vi "synth generation.vi"(8 "error in (no error)":errorcluster, 11 "Refnum in":T1) -> (0 "error out":errorcluster, 3 "Refnum out":T1)   [LabVIEW 2014]
uses:
  Controls/FPGA Reference.ctl
  Controls/ADSR State.ctl
  Controls/Application Data.vi
  <vilib>/Utility/error.llb/Error Cluster From Error Code.vi
  <vilib>/rvi/errors/niLvFpgaAdjustHostInterfaceError.vi
  <vilib>/rvi/interface/nirviMethod/nirviMethod.xnode
  <vilib>/FPGAPlugInAG/Dynamic/niLvFpga_WriteFifo_Dynamic.vi
  <vilib>/rvi/errors/niLvFpgaMergeErrorWithErrorCode.vi
panel:
  in  "Attack (ms) 2":dbl=1000.0
  in  "Max. Amplitude (V) 2":dbl(slide)=0.7993311036789298 scale=0.0..1.0
  in  "Sustain  2":dbl=0.6
  in  "Decay (ms) 2":dbl=300.0
  in  "Sustain 2":dbl=300.0
  in  "Release":dbl=300.0
  out "Gain2":dbl
  out "Gain Graph 2":dbl(graph)
  out "Waveform Chart":dbl[](graph)
  in  "Y":dbl[](array[numeric])
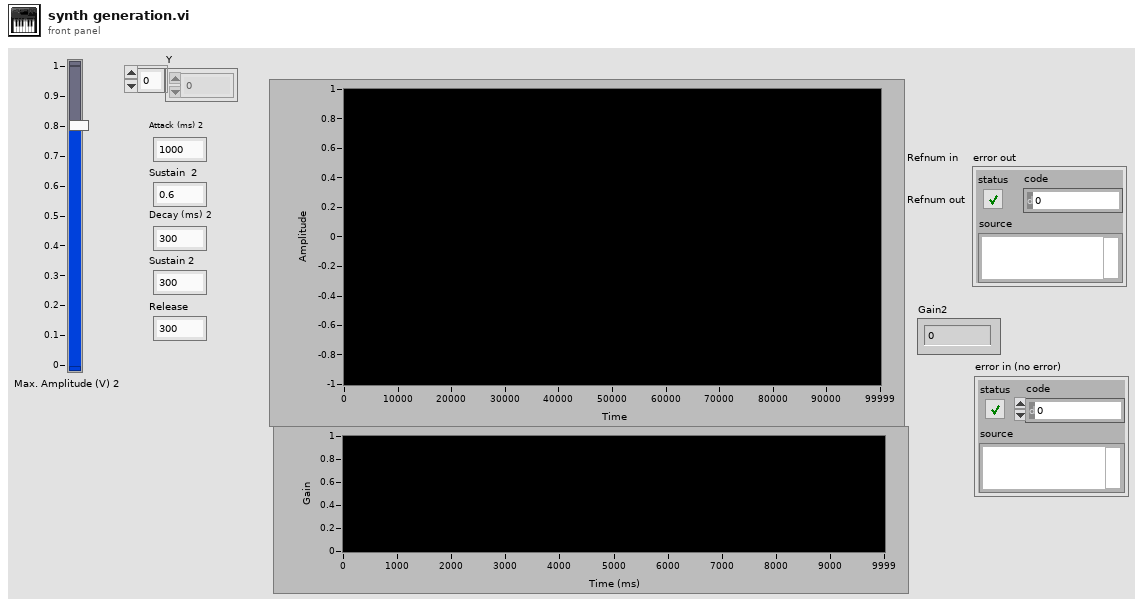
[diagram p1: front panel]
types:
  T1 = typedef "FPGA Reference.ctl" = refnum<k20>
  T2 = typedef "ADSR State.ctl" = enum16{"Attack", "Decay", "Sustain", "Release", "Idle"}
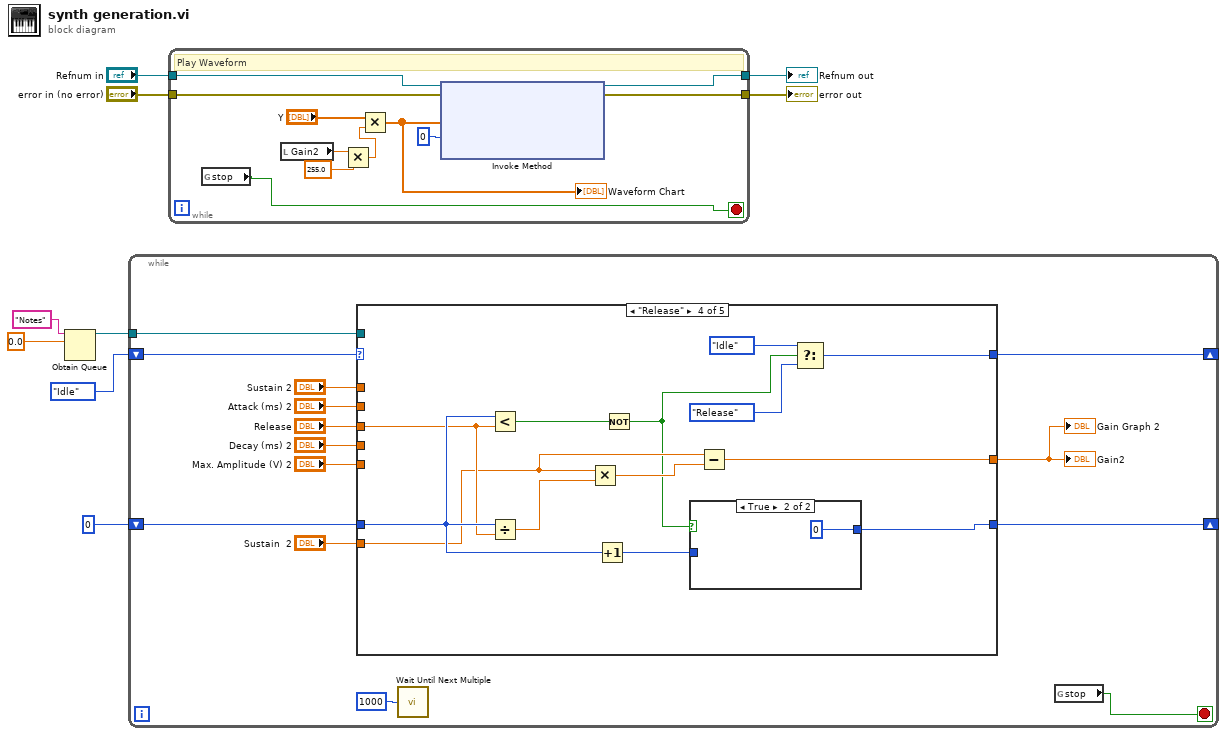
[diagram p0: block diagram]
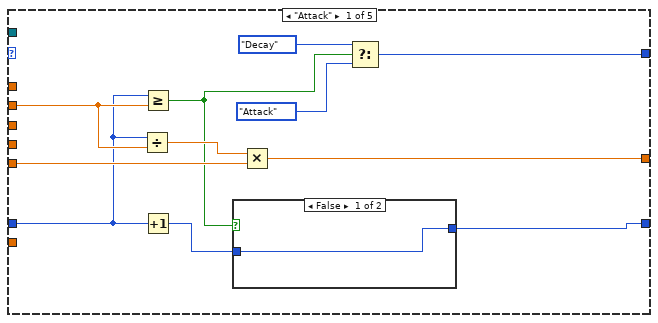
[diagram p2: hidden frame]
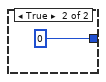
[diagram p3: hidden frame]
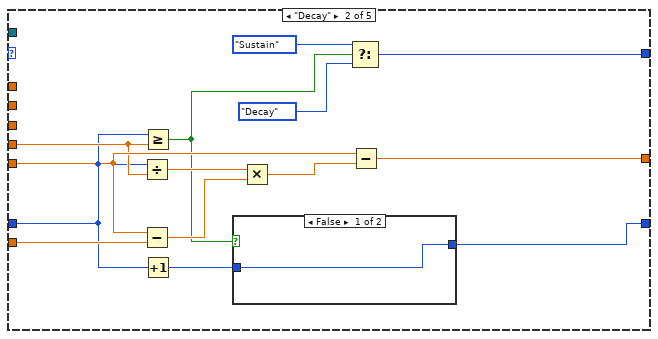
[diagram p4: hidden frame]
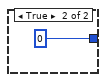
[diagram p5: hidden frame]
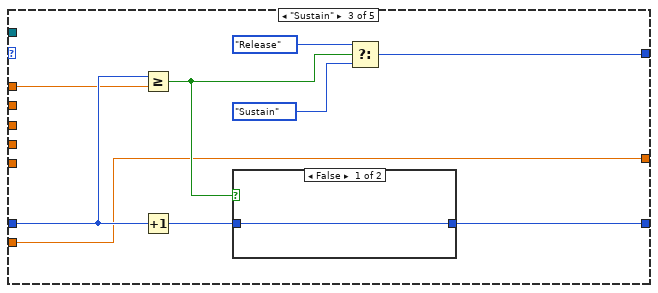
[diagram p6: hidden frame]
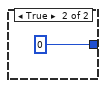
[diagram p7: hidden frame]
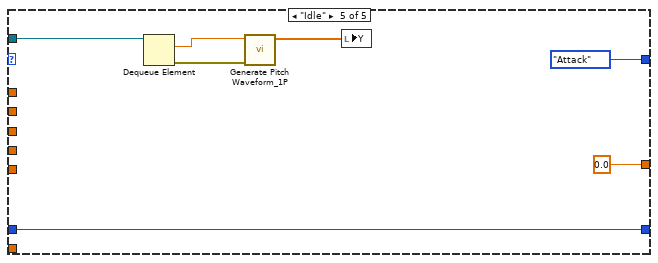
[diagram p9: hidden frame]
diagram:
  n1 = Obtain Queue(name (unnamed)="Notes", element data type=0.0) -> (queue out=w5:refnum<queue>)  [unwired: 3 in, 2 out]
  n2 = while {
    shift-right: [w16] -> _
    shift-left: ADSR_State."Idle" -> [w23]
    shift-right: [w13] -> _
    shift-left: 0 -> [w14]
    tunnel: w5 -> [w11]
    stop <- w10 stop-if-true
    n3 = case shown="\"Release\"" w23 {
      tunnel: "Sustain  2" -> [_ w50 w53 w69 _]
      tunnel: "Max. Amplitude (V) 2" -> [w33 w47 _ _ _]
      tunnel: "Attack (ms) 2" -> [w28 _ _ _ _]
      tunnel: "Decay (ms) 2" -> [_ w41 _ _ _]
      tunnel: "Sustain 2" -> [_ _ w54 _ _]
      tunnel: "Release" -> [_ _ _ w72 _]
      tunnel: w14 -> [w26 w39 w55 w73 w84]
      tunnel: [w32 w45 w53 w68 0.0 ("Sustain (%) 2")] -> w12
      tunnel: [w29 w42 w57 w67 ADSR_State."Attack"] -> w16
      tunnel: [w25 w37 w60 w75 w84] -> w13
      tunnel: w11 -> [_ _ _ _ w79]
      frame "Attack" {
        n4 = Divide(x=w26, y=w28) -> (x/y=w34:dbl)
        n5 = Greater Or Equal?(x=w26, y=w28) -> (x >= y?=w24:bool)
        n6 = Increment(x=w26) -> (x+1=w27:i32)
        n7 = case shown="False" w24 {
          tunnel: w27 -> [w35 _]
          tunnel: [w35 0] -> w25
          frame False {
          }
          frame True {
          }
        }
        n8 = Multiply(x=w34, y=w33) -> (x*y=w32:dbl)
        n9 = Select(t=ADSR_State."Decay", s=w24, f=ADSR_State."Attack") -> (s? t:f=w29:T2)
      }
      frame "Decay" {
        n10 = Divide(x=w39, y=w41) -> (x/y=w49:dbl)
        n11 = Subtract(x=w47, y=w50) -> (x-y=w48:dbl)
        n12 = Greater Or Equal?(x=w39, y=w41) -> (x >= y?=w40:bool)
        n13 = Increment(x=w39) -> (x+1=w38:i32)
        n14 = case shown="False" w40 {
          tunnel: w38 -> [w51 _]
          tunnel: [w51 0] -> w37
          frame False {
          }
          frame True {
          }
        }
        n15 = Multiply(x=w49, y=w48) -> (x*y=w46:dbl)
        n16 = Select(t=ADSR_State."Sustain", s=w40, f=ADSR_State."Decay") -> (s? t:f=w42:T2)
        n17 = Subtract(x=w47, y=w46) -> (x-y=w45:dbl)
      }
      frame "Sustain" {
        n18 = Greater Or Equal?(x=w55, y=w54) -> (x >= y?=w56:bool)
        n19 = Increment(x=w55) -> (x+1=w61:i32)
        n20 = case shown="False" w56 {
          tunnel: w61 -> [w62 _]
          tunnel: [w62 0] -> w60
          frame False {
          }
          frame True {
          }
        }
        n21 = Select(t=ADSR_State."Release", s=w56, f=ADSR_State."Sustain") -> (s? t:f=w57:T2)
      }
      frame "Release" {
        n22 = Less?(x=w73, y=w72) -> (x < y?=w74:bool)
        n23 = Divide(x=w73, y=w72) -> (x/y=w71:dbl)
        n24 = Multiply(x=w69, y=w71) -> (x*y=w70:dbl)
        n25 = Increment(x=w73) -> (x+1=w76:i32)
        n26 = Not(x=w74) -> (.not. x?=w64:bool)
        n27 = case shown="True" w64 {
          tunnel: w76 -> [w77 _]
          tunnel: [w77 0] -> w75
          frame False {
          }
          frame True {
          }
        }
        n28 = Subtract(x=w69, y=w70) -> (x-y=w68:dbl)
        n29 = Select(t=ADSR_State."Idle", s=w64, f=ADSR_State."Release") -> (s? t:f=w67:T2)
      }
      frame "Idle" {
        n30 = Dequeue Element(queue=w79) -> (element=w82:dbl, error out=w80:errorcluster)  [unwired: 2 in, 2 out]
        n31 = call "Generate Pitch Waveform_1P.vi"("Error In"=w80, "Pitch Frequency"=w82) -> ("Pitch Waveform"=w83:dbl[])  [unwired: 8 in, 1 out]
        n32 = local write "Y"(w83) -> ()
      }
    }
    "Gain2" <- w12
    "Gain Graph 2" <- w12
    n33 = call "Wait Until Next Multiple"("Count(uSec)"=u32 1000) -> ()  [unwired: 1 out]
    n34 = global read "Application Data.vi" "stop"() -> (w10:bool)
  }
  n35 = while {
    tunnel: "Refnum in" -> [w94]
    tunnel: [w93] -> w2
    tunnel: [w92] -> w3
    tunnel: "error in (no error)" -> [w90]
    stop <- w89 stop-if-true
    # "Play Waveform"
    n36 = global read "Application Data.vi" "stop"() -> (w89:bool)
    n37 = local read "Gain2"() -> (w88:dbl)
    n38 = Multiply(x=w88, y=255.0) -> (x*y=w86:dbl)
    n39 = Multiply(x="Y", y=w86) -> (x*y=w96:dbl[])
    "Waveform Chart" <- w96
    n40 = xnode "Invoke Method"("FPGA VI Reference In"=w94, "error in"=w90, "Data"=w96, "Timeout (ms)"=0) -> ("FPGA VI Reference Out"=w92:T1, "error out"=w93:errorcluster)  [unwired: 1 out]
  }
  "Refnum out" <- w3
  "error out" <- w2
